vi "Front Panel.vi"(11 "GUI In":refnum<class "Common UI.lvclass">) -> ()   [LabVIEW 2015, in "Common UI.lvclass"]
uses:
  Common UI.lvclass
  Reusable/Xctls/Buffer/1D Control/1D Buffer.xctl
  Reusable/GUI/GUI.lvclass/GUI.ctl
  Reusable/Observer/Observer.lvclass/Observer.ctl
  Data/cPAS Data.lvclass
  Reusable/GUI/Accessors/Read RegEvent.vi
  Reusable/Observer/Read Data Queue.vi
  Reusable/Data/Read measTime.vi
  Data/Read dcVolts.vi
  Reusable/Data/Data.lvclass
panel:
  out "Power":cluster{"time":timestamp, "data":sgl[]}(xcontrol)
  in  "Filter DC":cluster{"On":u16, "Off":u16}
  out "timestamp":timestamp format="%<%H:%M:%S%2u>T"
  in  "Power":T1
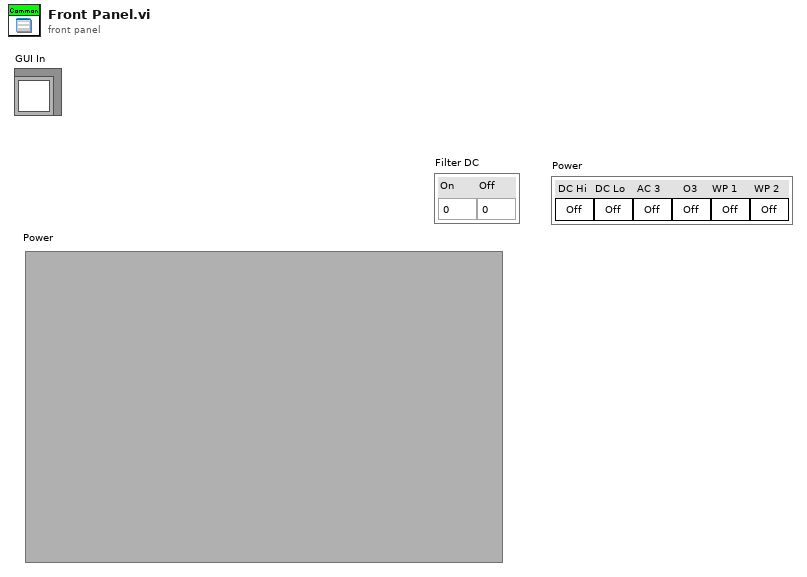
[diagram p1: front panel]
types:
  T1 = cluster{"DC Hi":bool, "DC Lo":bool, "AC 3":bool, "O3":bool, "WP 1":bool, "WP 2":bool}
  T2 = cluster{"24V":sgl, "+15V":sgl, "- 15V":sgl, "12V":sgl, "Aux Volt":sgl}
  T3 = cluster{"Array of UInt16[0]":u16, "Array of UInt16[1]":u16}
  T4 = cluster{"Array of Boolean[0]":bool, "Array of Boolean[1]":bool, "Array of Boolean[2]":bool, "Array of Boolean[3]":bool, "Array of Boolean[4]":bool, "Array of Boolean[5]":bool}
  T5 = cluster{"Time":timestamp, "Accessors:dcVolts":sgl[]}
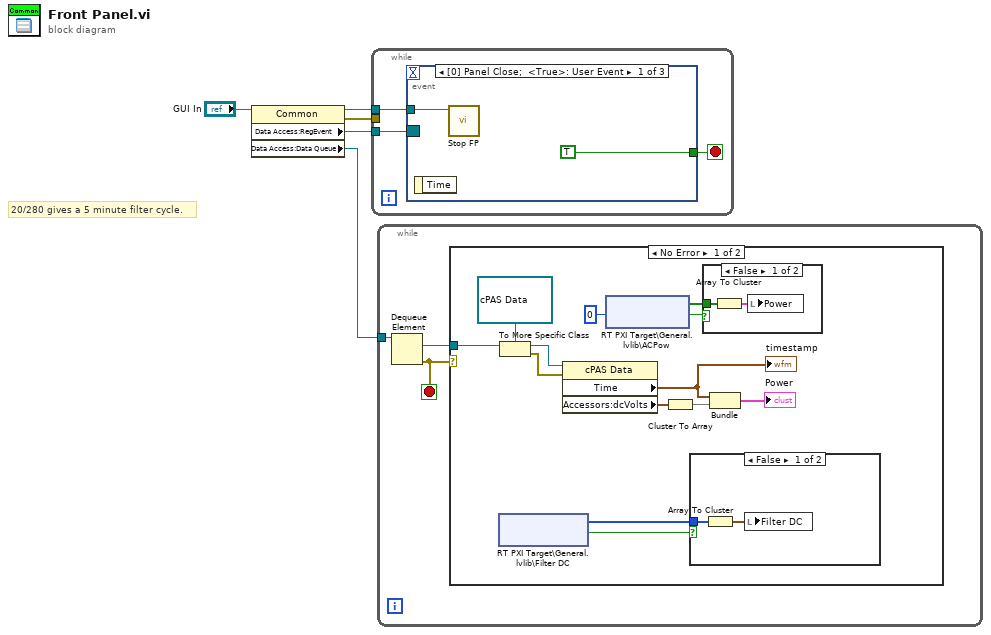
[diagram p0: block diagram]
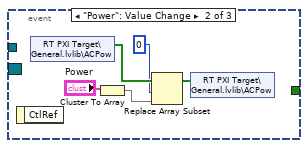
[diagram p5: hidden frame]
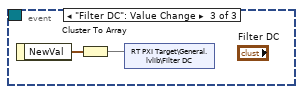
[diagram p6: hidden frame]
diagram:
  # "20/280 gives a 5 minute filter cycle."
  n1 = property class="Common"(reference="GUI In") -> (reference out=w3:refnum<class "Common UI.lvclass">, error out=w1:errorcluster, "Data Access:RegEvent"=w4:refnum<event-registration>, "Data Access:Data Queue"=w2:refnum<queue>)  [unwired: 1 in]
  n2 = while {
    tunnel: w4 -> [w7]
    tunnel: w3 -> [w6]
    tunnel: w1 -> [_]
    stop <- w8 stop-if-true
    n3 = event shown="[0] Panel Close;  <True>: User Event" {
      selector: w7 -> [_ _ _]
      dyn-events: _ -> [_ _ _]
      timeout: _ -> [_ _ _]
      tunnel: [TRUE _ _] -> w8
      tunnel: w6 -> [w9 _ _]
      event Panel Close; User Event {
        n4 = event-data() -> ()  [unwired: 1 in, 1 out]
        n5 = call-dynamic "Stop FP.vi"("GUI in"=w9) -> ()  [unwired: 9 in, 2 out]
      }
      event "Power": Value Change {
        n6 = event-data() -> ()  [unwired: 1 in, 1 out]
        n7 = shared-variable "RT PXI Target\\General.lvlib\\ACPow"() -> (w14:bool[])  [unwired: 1 in, 1 out]
        n8 = Cluster To Array(cluster="Power") -> (array=w13:bool[])
        n9 = Replace Array Subset(array=w14, new element=w13, index=0) -> (w12:bool[])
        n10 = shared-variable "RT PXI Target\\General.lvlib\\ACPow"(w12) -> ()  [unwired: 1 in, 1 out]
      }
      event "Filter DC": Value Change {
        n11 = event-data() -> ("NewVal"=w17:cluster{"On":u16, "Off":u16})  [unwired: 1 in]
        n12 = Cluster To Array(cluster=w17) -> (array=w16:u16[])
        n13 = shared-variable "RT PXI Target\\General.lvlib\\Filter DC"(w16) -> ()  [unwired: 1 in, 1 out]
      }
    }
  }
  n14 = while {
    tunnel: w2 -> [w20]
    stop <- w19 stop-if-true
    n15 = Dequeue Element(queue=w20) -> (element=w18:refnum<data-value>, error out=w19:errorcluster)  [unwired: 2 in, 2 out]
    n16 = case shown="No Error" w19 {
      tunnel: w18 -> [w30 _]
      frame No Error {
        n17 = shared-variable "RT PXI Target\\General.lvlib\\Filter DC"() -> (w21:u16[], w22:bool)  [unwired: 2 in, 1 out]
        n18 = To More Specific Class(target class=refnum<data-value> refnum ("DVR"), reference=w30) -> (specific class reference=w28:refnum<data-value>, error out=w25:errorcluster)  [unwired: 1 in]
        n19 = property class="cPAS Data"(reference=w28, error in=w25) -> ("Time"=w23:timestamp, "Accessors:dcVolts"=w24:T2)  [unwired: 2 out]
        "timestamp" <- w23
        n20 = shared-variable "RT PXI Target\\General.lvlib\\ACPow"(0 ("ms timeout (0)")) -> (w31:bool[], w32:bool)  [unwired: 1 in, 1 out]
        n21 = Cluster To Array(cluster=w24) -> (array=w27:sgl[])
        n22 = case shown="False" w22 {
          tunnel: w21 -> [w35 _]
          frame False {
            n23 = Array To Cluster(array=w35) -> (cluster=w34:T3)
            n24 = local write "Filter DC"(w34) -> ()
          }
          frame True {
          }
        }
        n25 = case shown="False" w32 {
          tunnel: w31 -> [w37 _]
          frame False {
            n26 = Array To Cluster(array=w37) -> (cluster=w36:T4)
            n27 = local write "Power"(w36) -> ()
          }
          frame True {
          }
        }
        n28 = Bundle("Time"=w23, "Accessors:dcVolts"=w27) -> (→"Power":T5)  [unwired: 1 in]
      }
      frame Error {
      }
    }
  }
